vi "RSZVB Linearity Deviation Manual.vi"(6 "Constant (0.0 dB)":dbl format="%^.3e", 7 "Electrical Length (0.0 m)":dbl format="%^.3e", 8 "error in (no error)":errorcluster {"code" format="%.0x"}, 9 "Slope (0.0 dB/MHz)":dbl format="%^.3e", 10 "Channel (1)":i32=1, 11 "VISA session":refnum<visa-resource-name>) -> (0 "error out":errorcluster {"code" format="%.0x"}, 3 "dup VISA session":refnum<visa-resource-name>)   [LabVIEW 2011]
doc: "This VI is used for manual entry of the correction factors. \n\nNote(s):\n\n(1) Electrical length is available if the active trace format is Phase or Unwrapped Phase, or if a mixer delay is measured.\n\nRemote-control command(s):\nCALCulate<Chn>:LDEViation:SLOPe\nCALCulate<Chn>:LDEViation:CONStant\nCALCulate<Chn>:LDEViation:ELENgth"
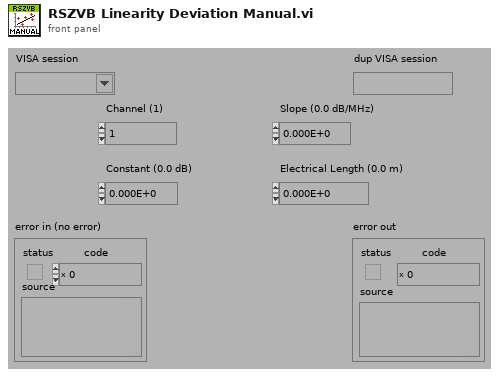
[diagram p1: front panel]
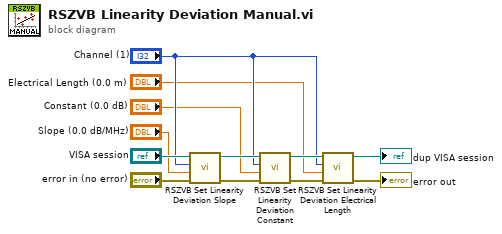
[diagram p0: block diagram]
diagram:
  n1 = call "RSZVB Set Linearity Deviation Slope.vi"("error in (no error)"="error in (no error)", "Slope (0.0 dB/MHz)"="Slope (0.0 dB/MHz)", "Channel (1)"="Channel (1)", "VISA session"="VISA session") -> ("error out"=w11:errorcluster, "dup VISA session"=w8:refnum<visa-resource-name>)  [unwired: 6 in]
  n2 = call "RSZVB Set Linearity Deviation Constant.vi"("error in (no error)"=w11, "Constant (0.0 dB)"="Constant (0.0 dB)", "Channel (1)"="Channel (1)", "VISA session"=w8) -> ("error out"=w10:errorcluster, "dup VISA session"=w7:refnum<visa-resource-name>)  [unwired: 6 in]
  n3 = call "RSZVB Set Linearity Deviation Electrical Length.vi"("error in (no error)"=w10, "Electrical Length (0.0)"="Electrical Length (0.0 m)", "Channel (1)"="Channel (1)", "VISA session"=w7) -> ("error out"=→"error out":errorcluster, "dup VISA session"=→"dup VISA session":refnum<visa-resource-name>)  [unwired: 6 in]
